vi "7.2.1.vi"() -> ()   [LabVIEW 2018]
panel:
  in  "b":string
  in  "a":bool
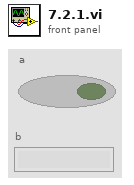
[diagram p1: front panel]
types:
  T1 = enum8{"Enabled", "Disabled", "Disabled and Grayed Out"}
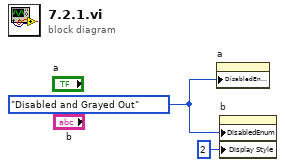
[diagram p0: block diagram]
diagram:
  w2 = T1."Disabled and Grayed Out" ("비활성화")
  n1 = property on="a" class="Bool (엄격한)"("DisabledEnum"=w2) -> ()  [unwired: 2 in, 2 out]
  n2 = property on="b" class="Str"("DisabledEnum"=w2, "Display Style"=u32 2 ("디스플레이 스타일")) -> ()  [unwired: 2 in, 2 out]
